vi "Write v_norm.vi"(8 "error in (no error)":errorcluster, 10 "v_norm":dbl, 11 "Robot in":refnum<class "Robot.lvclass">) -> (0 "error out":errorcluster, 3 "Robot out":refnum<class "Robot.lvclass">)   [LabVIEW 2020, in "Robot.lvclass"]
uses:
  Robot.lvclass
  Robot.lvclass/Robot.ctl
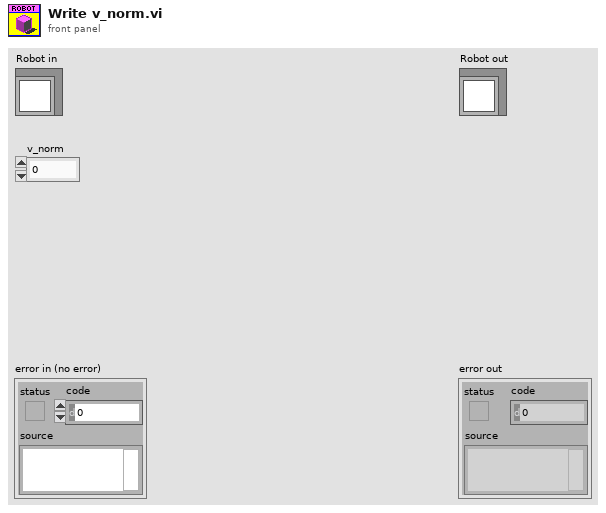
[diagram p1: front panel]
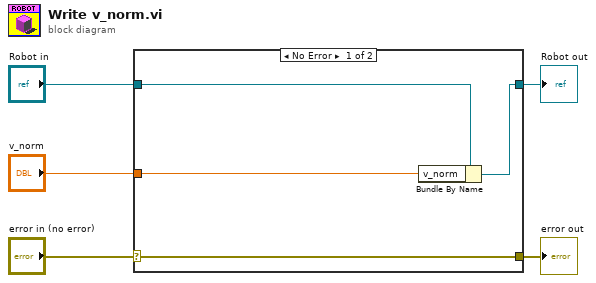
[diagram p0: block diagram]
diagram:
  n1 = case shown="No Error" "error in (no error)" {
    selector: "error in (no error)" -> [w9 w10]
    tunnel: [w9 w10] -> w4
    tunnel: [w7 w11] -> w2
    tunnel: "Robot in" -> [w8 w11]
    tunnel: "v_norm" -> [w6 _]
    frame No Error {
      n2 = Bundle By Name(cluster=w8, "v_norm"=w6) -> (w7:refnum<class "Robot.lvclass">)
    }
    frame Error {
    }
  }
  "error out" <- w4
  "Robot out" <- w2
